vi "Add Rx Label.vi"(6 "create channels":T1, 8 "error in":errorcluster, 9 "SDI value":T3=-1 items=["All"=-1, "0 (b00)"=0, "1 (b01)"=1, "2 (b10)"=2, "3 (b11)"=3], 10 "label value":u32, 11 "port ref":T2 format="%.0x") -> (0 "error out":errorcluster, 2 "label ref":T2 format="%.0x", 3 "port ref out":T2 format="%.0x")   [LabVIEW 2020, in "Ballard ARINC 429 Scripting.lvlib"]
uses:
  Ballard ARINC 429 Scripting.lvlib
  Shared/SDI.ctl
  <vilib>/NI VeriStand/Custom Device API/Custom Device Item Ref.ctl
  Shared/Label Properties.ctl
  Shared/Label.ctl
  <vilib>/NI VeriStand/Custom Device API/Custom Device Channel.ctl
  <vilib>/NI VeriStand/Custom Device API/Custom Device Channel Type.ctl
  Constants.vi
  ARINC 429/Constants.vi
  <vilib>/NI VeriStand/Custom Device API/Custom Device API.lvlib
  ARINC 429/ARINC 429 Scripting.lvlib
  Import/ARINC 429 Import.lvlib
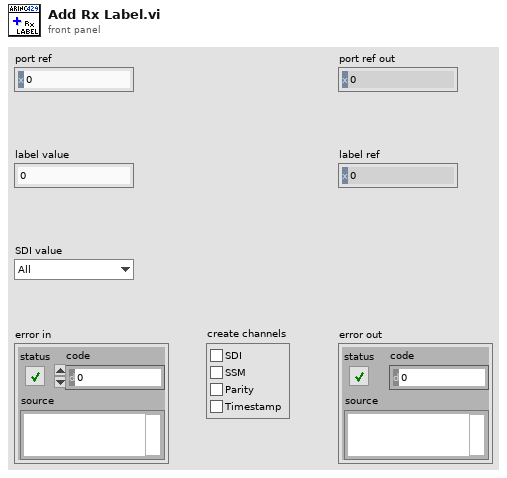
[diagram p1: front panel]
types:
  T1 = cluster{"SDI":bool, "SSM":bool, "Parity":bool, "Timestamp":bool}
  T2 = typedef "Custom Device API.lvlib/Custom Device Item Ref.ctl" = u64
  T3 = typedef "SDI.ctl" = i32
  T4 = typedef "Direction.ctl" = enum16{"Rx", "Tx"}
  T5 = typedef "Label Properties.ctl" = cluster{"label (Dec)":T6, "SDI value":u8, "SDI enabled":bool}
  T6 = typedef "Label.ctl" = u8
  T7 = typedef "Custom Device API.lvlib/Custom Device Channel.ctl" = cluster{"Type":T8, "Units":string, "Default Value":dbl, "Faultable":bool, "Scalable":bool}
  T8 = typedef "Custom Device API.lvlib/Custom Device Channel Type.ctl" = enum16{"Input", "Output"}
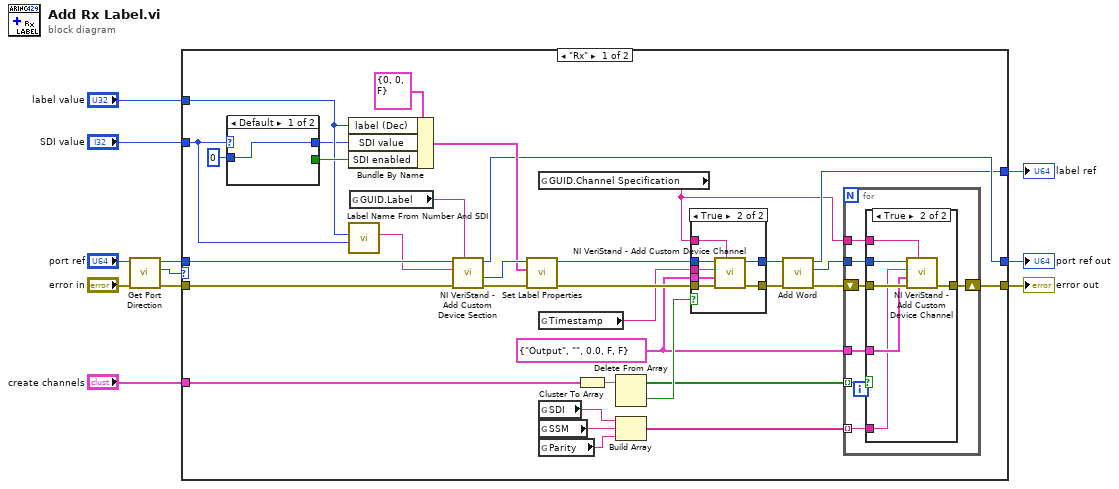
[diagram p0: block diagram]
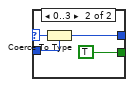
[diagram p4: hidden frame]
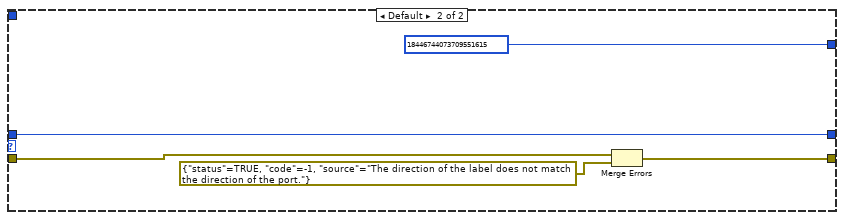
[diagram p5: hidden frame]
diagram:
  n1 = call "Get Port Direction.vi"("error in"="error in", "port ref in"="port ref") -> ("error out"=w8:errorcluster, "direction"=w1:T4, "port ref out"=w9:T2)  [unwired: 7 in]
  n2 = case shown="\"Rx\"" w1 {
    tunnel: w9 -> [w36 w77]
    tunnel: w8 -> [w35 w75]
    tunnel: [w32 w77] -> w7
    tunnel: "label value" -> [w29 _]
    tunnel: "SDI value" -> [w27 _]
    tunnel: "create channels" -> [w26 _]
    tunnel: [w23 T2 18446744073709551615 ("label ref out")] -> w3
    tunnel: [w21 w74] -> w2
    frame "Rx" {
      w17 = T7 {"Type"=enum."Output", "Units"="", "Default Value"=0.0, "Faultable"=FALSE, "Scalable"=FALSE} ("Channel")
      n3 = case shown="Default" w27 {
        selector: w27 -> [_ w72]
        tunnel: [w68 w69] -> w28
        tunnel: u8 0 ("SDI value") -> [w68 w71]
        tunnel: [_ TRUE] -> w33
        frame Default {
        }
        frame 0..3 {
          n4 = Coerce To Type(0:w72, 1:w71) -> (2:w69:u8)
        }
      }
      n5 = Bundle By Name(cluster=T5 {"label (Dec)"=0, "SDI value"=0, "SDI enabled"=FALSE} ("label properties"), "label (Dec)"=w29, "SDI value"=w28, "SDI enabled"=w33) -> (w37:T5)
      n6 = call "Label Name From Number And SDI.vi"("SDI value"=w27, "label (Dec)"=w29) -> ("label name"=w30:string)  [unwired: 9 in]
      n7 = global read "Constants.vi" "GUID.Label"() -> (w39:string)
      n8 = call <vilib>:"NI VeriStand - Add Custom Device Section.vi"("GUID (Default Section)"=w39, "error in (no error)"=w35, "Section Name"=w30, "Parent Ref in"=w36) -> ("error out"=w41:errorcluster, "Section Ptr"=w40:T2, "Parent Ref out"=w32:T2)  [unwired: 4 in, 1 out]
      n9 = call "Set Label Properties.vi"("error in"=w41, "label properties"=w37, "label ref"=w40) -> ("error out"=w42:errorcluster, "label ref out"=w31:T2)  [unwired: 7 in]
      n10 = global read "Constants.vi" "GUID.Channel Specification"() -> (w18:string)
      n11 = global read "Constants.vi" "Timestamp"() -> (w12:string)
      n12 = global read "Constants.vi" "SDI"() -> (w15:string)
      n13 = global read "Constants.vi" "SSM"() -> (w16:string)
      n14 = global read "Constants.vi" "Parity"() -> (w14:string)
      n15 = Cluster To Array(cluster=w26) -> (array=w25:bool[])
      n16 = Delete From Array(array=w25) -> (deleted portion=w24:bool, array with subset deleted=w20:bool[])  [unwired: 2 in]
      n17 = Build Array(w15, w16, w14) -> (w13:string[])
      n18 = case shown="True" w24 {
        tunnel: [w60 w67] -> w44
        tunnel: [w59 w66] -> w43
        tunnel: w42 -> [w59 w65]
        tunnel: w31 -> [w60 w64]
        tunnel: w18 -> [_ w63]
        tunnel: w17 -> [_ w62]
        tunnel: w12 -> [_ w61]
        frame False {
        }
        frame True {
          n19 = call <vilib>:"NI VeriStand - Add Custom Device Channel.vi"("GUID (Default Channel)"=w63, "error in (no error)"=w65, "Channel"=w62, "Channel Name"=w61, "Parent Ref in"=w64) -> ("error out"=w66:errorcluster, "Parent Ref out"=w67:T2)  [unwired: 3 in, 2 out]
        }
      }
      n20 = call "Add Word.vi"("error in"=w43, "label ref"=w44) -> ("error out"=w22:errorcluster, "word ref"=w19:T2, "label ref out"=w23:T2)  [unwired: 6 in, 1 out]
      n21 = for {
        shift-right: [w50] -> w21
        shift-left: w22 -> [w49]
        tunnel: w20 -> [w51] mode=indexing
        tunnel: w19 -> [w48]
        tunnel: w18 -> [w47]
        tunnel: w17 -> [w46]
        tunnel: w13 -> [w45] mode=indexing
        n22 = case shown="True" w51 {
          tunnel: [w52 w58] -> w50
          tunnel: w49 -> [w52 w57]
          tunnel: w48 -> [_ w54]
          tunnel: w47 -> [_ w56]
          tunnel: w46 -> [_ w55]
          tunnel: w45 -> [_ w53]
          frame False {
          }
          frame True {
            n23 = call <vilib>:"NI VeriStand - Add Custom Device Channel.vi"("GUID (Default Channel)"=w56, "error in (no error)"=w57, "Channel"=w55, "Channel Name"=w53, "Parent Ref in"=w54) -> ("error out"=w58:errorcluster)  [unwired: 3 in, 3 out]
          }
        }
      }
    }
    frame Default {
      n24 = Merge Errors(w75, errorcluster {"status"=TRUE, "code"=-1, "source"="The direction of the label does not match the direction of the port."} ("error in")) -> (w74:errorcluster)
    }
  }
  "label ref" <- w3
  "error out" <- w2
  "port ref out" <- w7
